vi "read_vacuum.vi"() -> (0 "Vac Remote":bool, 1 "Atm Exhaust":bool, 2 "Vac Exhaust":bool)   [LabVIEW 2011]
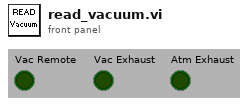
[diagram p1: front panel]
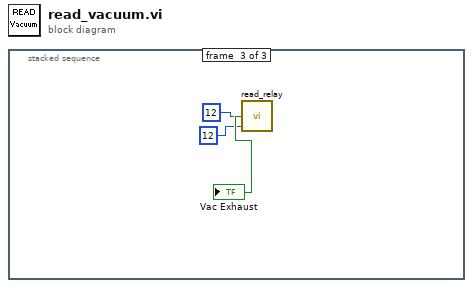
[diagram p0: block diagram]
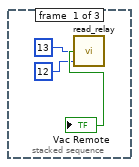
[diagram p2: hidden frame]
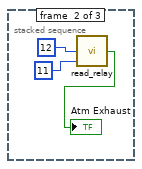
[diagram p3: hidden frame]
diagram:
  n1 = stacked-sequence {
    frame #0 {
      n2 = call "read_relay.vi"("Relay"=12, "Slot"=13) -> ("Relay Status"=→"Vac Remote":bool)  [unwired: 1 out]
    }
    frame #1 {
      n3 = call "read_relay.vi"("Relay"=11, "Slot"=12) -> ("Relay Status"=→"Atm Exhaust":bool)  [unwired: 1 out]
    }
    frame #2 {
      n4 = call "read_relay.vi"("Relay"=12, "Slot"=12) -> ("Relay Status"=→"Vac Exhaust":bool)  [unwired: 1 out]
    }
  }
